vi "Write Cell String.vi"(0 "Report Ref In":T1, 1 "Row Index":i32, 2 "Column Index":i32, 3 "error in (no error)":errorcluster, 4 "Value":string) -> (5 "Report Ref Out":T1, 6 "error out":errorcluster)   [LabVIEW 2026, in "XCel Report Engine.lvlib"]
uses:
  XCel Report Engine.lvlib
  Controls/Report Ref.ctl
  C:/Users/m.santucci/Documents/ChatGPT/LV_REPORT_ENGINE/.net/src/XCelReportEngine/bin/Release/net48/XCelReportEngine.dll
  .net/src/XCelReportEngine/bin/Release/net48/XCelReportEngine.dll
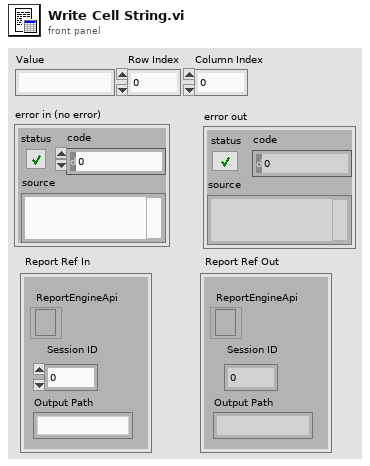
[diagram p1: front panel]
types:
  T1 = typedef "XCel Report Engine.lvlib/Report Ref.ctl" = cluster{"Session ID":i32, "Output Path":string, "ReportEngineApi":refnum<k24>}
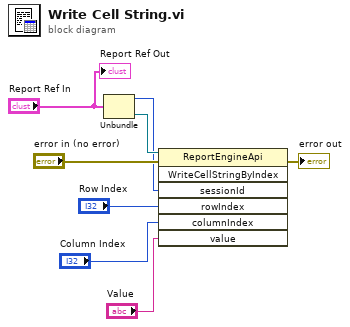
[diagram p0: block diagram]
diagram:
  n1 = Unbundle("Report Ref In") -> ("Session ID"=w4:i32, "ReportEngineApi"=w7:refnum<k24>)  [unwired: 1 out]
  n2 = invoke class="ReportEngineApi" method="WriteCellStringByIndex"(reference=w7, error in="error in (no error)", "sessionId"=w4, "rowIndex"="Row Index", "columnIndex"="Column Index", "value"="Value") -> (error out=→"error out":errorcluster)  [unwired: 1 in, 6 out]
  "Report Ref Out" <- "Report Ref In"
